vi "magnet_ps_pd_get.vi"(8 "error in (no error)":errorcluster, 10 "Wait untill read (S)":dbl=0.1, 11 "VISA resource name":refnum<visa-resource-name>) -> (0 "error out":errorcluster, 3 "VISA resource name out":refnum<visa-resource-name>)   [LabVIEW 2019]
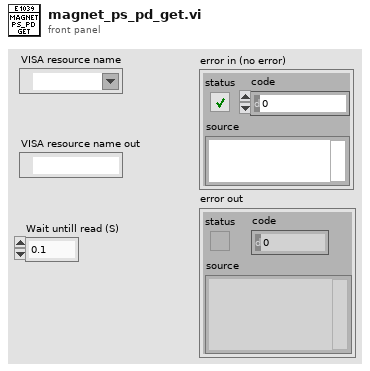
[diagram p1: front panel]
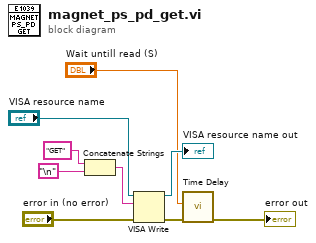
[diagram p0: block diagram]
diagram:
  n1 = Concatenate Strings("GET" ("string"), "\n") -> (w6:string)
  n2 = VISA Write(VISA resource name="VISA resource name", write buffer=w6, error in (no error)="error in (no error)") -> (VISA resource name out=→"VISA resource name out":refnum<visa-resource-name>, error out=w8:errorcluster)  [unwired: 1 out]
  n3 = call "Time Delay"("error in (no error)"=w8, "Delay Time (s)"="Wait untill read (S)") -> ("error out"=→"error out":errorcluster)  [unwired: 9 in]
